vi "TestSorting.vi"() -> ()   [LabVIEW 2009]
panel:
  out "A3":i32[](array[numeric])
  out "A2":i32[](array[numeric])
  out "A1":i32[](array[numeric])
  in  "Setup.ImChannels":u8=2
  out "Status.Bad PMTData":bool
  out "Status.DownsampleDone":bool
  out "Debug.PMT Array":i32[](array[numeric])
  out "Scan.Samples":u32
  in  "Scan.TotalSamples":u32
  in  "Setup.Channels":u8=2
  in  "Setup.PMT Timeout":u32=200000
  in  "AOD.ThrowawaySamples":u16=40
  in  "AOD.BlankSamples":u16=40
  in  "Control.Abort":bool
  in  "Setup.Downsample":u32=80
  in  "Scan.Motion Increment":u32
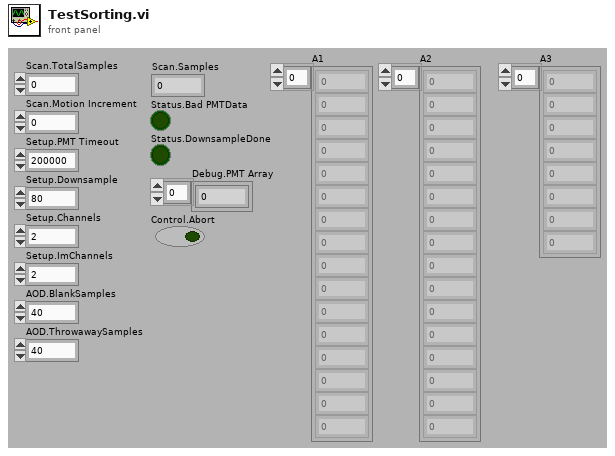
[diagram p1: front panel]
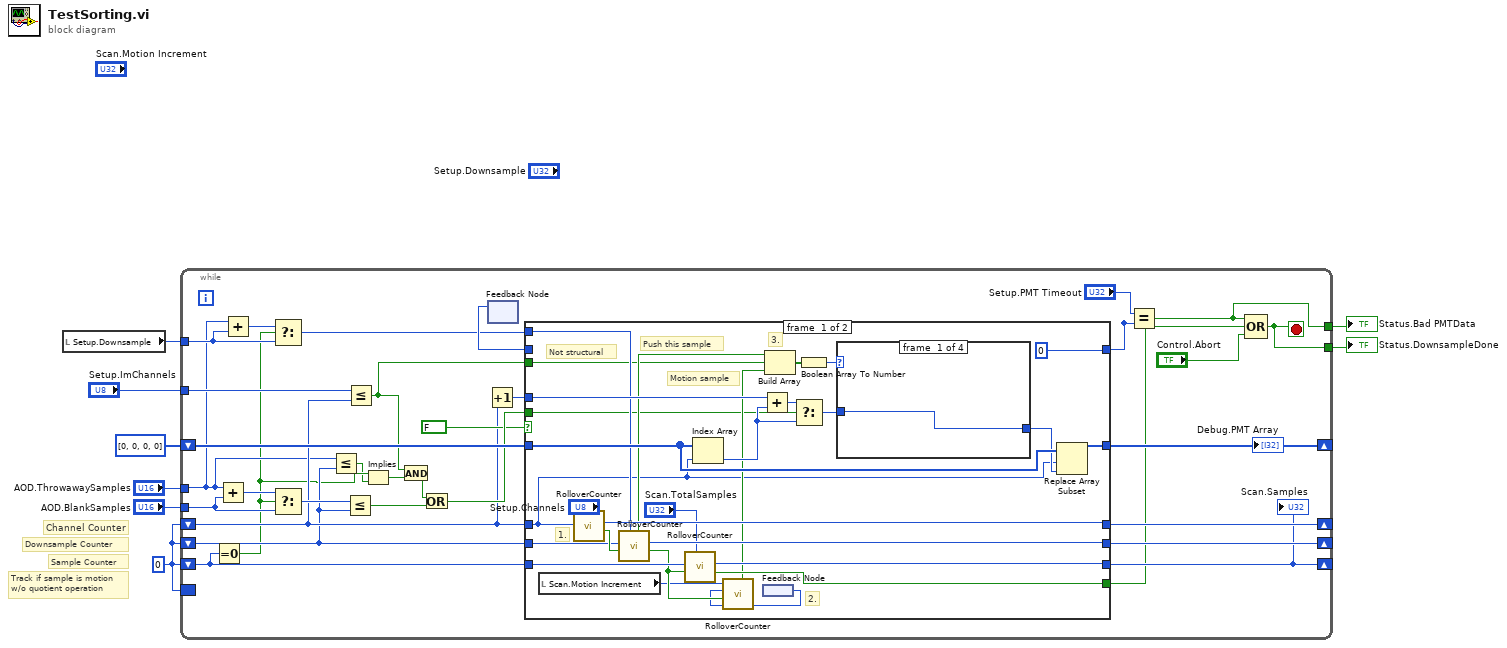
[diagram p0: block diagram]
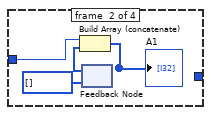
[diagram p2: hidden frame]
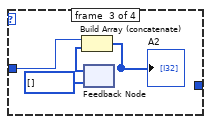
[diagram p3: hidden frame]
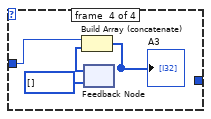
[diagram p4: hidden frame]
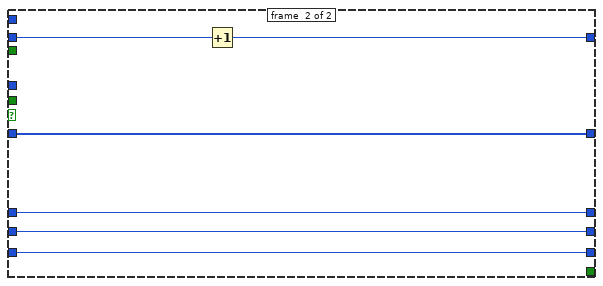
[diagram p5: hidden frame]
diagram:
  w2 = u32 0
  # "Track if sample is motion\nw/o quotient operation"
  # "Sample Counter"
  # "Downsample Counter"
  # "Channel Counter"
  n1 = local read "Setup.Downsample"() -> (w8:u32)
  n2 = while {
    shift-right: [w29] -> _
    shift-left: w2 -> [w35]
    tunnel: "AOD.BlankSamples" -> [w40]
    tunnel: "AOD.ThrowawaySamples" -> [w14]
    tunnel: w8 -> [w37]
    shift-right: [w31] -> _
    shift-left: w2 -> [w15]
    shift-right: [w28] -> _
    shift-left: i32[] [0, 0, 0, 0] -> [w36]
    shift-right: [w32] -> _
    shift-left: w2 -> [w16]
    tunnel: [w26] -> w4
    tunnel: [w25] -> w3
    tunnel: "Setup.ImChannels" -> [w23]
    border: w2 -> [_]
    stop <- w26 stop-if-true
    n3 = Equal To 0?(x=w35) -> (x = 0?=w10:bool)
    n4 = Add(x=w14, y=w40) -> (x+y=w39:u16)
    n5 = Add(x=w14, y=w37) -> (x+y=w38:u32)
    n6 = Select(t=w38, s=w10, f=w37) -> (s? t:f=w30:u32)
    n7 = Select(t=w39, s=w10, f=w40) -> (s? t:f=w24:u16)
    n8 = Less Or Equal?(x=w14, y=w15) -> (x <= y?=w9:bool)
    n9 = Less Or Equal?(x=w24, y=w15) -> (x <= y?=w22:bool)
    n10 = Less Or Equal?(x=w23, y=w16) -> (x <= y?=w12:bool)
    n11 = Implies(1:w9, 2:w10) -> (0:w11:bool)
    n12 = And(x=w12, y=w11) -> (x .and. y?=w13:bool)
    n13 = Or(x=w13, y=w22) -> (x .or. y?=w21:bool)
    n14 = Increment(x=w16) -> (x+1=w17:u32)
    n15 = feedback #1() -> (w34:i16)  [unwired: 1 in]
    n16 = case shown="False" FALSE {
      tunnel: w17 -> [w68 _]
      tunnel: w36 -> [w66 w88]
      tunnel: [w67 w88] -> w28
      tunnel: w16 -> [w44 w85]
      tunnel: w15 -> [w54 w84]
      tunnel: w35 -> [w63 w83]
      tunnel: [i16 0 w87] -> w33
      tunnel: w34 -> [_ w86]
      tunnel: [w64 w85] -> w32
      tunnel: [w59 w84] -> w31
      tunnel: [w62 w83] -> w29
      tunnel: w30 -> [w50 _]
      tunnel: [w61 _] -> w27
      tunnel: w12 -> [w46 _]
      tunnel: w21 -> [w45 _]
      frame #0 {
        # "Motion sample"
        # "Not structural"
        # "Push this sample"
        # "3."
        # "2."
        # "1."
        n17 = local read "Scan.Motion Increment"() -> (w41:u32)
        n18 = call "RolloverCounter.vi"("RolloverNum"="Setup.Channels", "In"=w44) -> ("Rollover"=w60:bool, "Count"=w64:u32)  [unwired: 7 in, 1 out]
        n19 = call "RolloverCounter.vi"("RolloverNum"=w50, "Increment"=w60, "In"=w54) -> ("Rollover"=w57:bool, "Count"=w59:u32, "Last"=w47:bool)  [unwired: 6 in]
        n20 = call "RolloverCounter.vi"("RolloverNum"="Scan.TotalSamples", "Increment"=w57, "In"=w63) -> ("Rollover"=w61:bool, "Count"=w62:u32)  [unwired: 6 in, 1 out]
        n21 = Index Array(array=w66, index=w44) -> (element=w52:i32)
        n22 = Add(x=w68, y=w52) -> (x+y=w53:u32)
        n23 = feedback #2() -> (w42:u32)
        n24 = call "RolloverCounter.vi"("RolloverNum"=w41, "Increment"=w57, "In"=w42) -> ("Count"=w43:u32, "Last"=w49:bool)  [unwired: 6 in, 1 out]
        n25 = Build Array(w47, w46, w49) -> (w56:bool[])
        n26 = Select(t=w53, s=w45, f=w52) -> (s? t:f=w51:u32)
        n27 = Boolean Array To Number(Boolean array=w56) -> (number=w55:u8)
        n28 = case shown="3, 7" w55 {
          tunnel: [w70 _ _ _] -> w65
          tunnel: w51 -> [w70 w74 w76 w80]
          frame #0 {
          }
          frame #1 {
            n29 = feedback #3(i32[] []) -> (w72:u32[])
            n30 = Build Array (concatenate)(w74, w72) -> (w73:u32[])
            "A1" <- w73
          }
          frame #2 {
            n31 = feedback #4(i32[] []) -> (w77:u32[])
            n32 = Build Array (concatenate)(w76, w77) -> (w78:u32[])
            "A2" <- w78
          }
          frame #3 {
            n33 = feedback #5(i32[] []) -> (w81:u32[])
            n34 = Build Array (concatenate)(w80, w81) -> (w82:u32[])
            "A3" <- w82
          }
        }
        n35 = Replace Array Subset(array=w66, new element=w65, index=w44) -> (w67:i32[])
      }
      frame #1 {
        n36 = Increment(x=w86) -> (x+1=w87:i16)
      }
    }
    "Debug.PMT Array" <- w28
    "Scan.Samples" <- w29
    n37 = Equal?(x="Setup.PMT Timeout", y=w33) -> (x = y?=w25:bool)
    n38 = Compound Arithmetic op=OR(w25, w27, "Control.Abort") -> (w26:bool)
  }
  "Status.DownsampleDone" <- w4
  "Status.Bad PMTData" <- w3
